vi "Строка параметров в I8 (SubVI).vi"(8 "Строка чисел параметров мишеней":string) -> (9 "Остаток строки":string, 16 "Кластер чисел типа I8":T1)   [LabVIEW 2013]
doc: "Преобразование строки с числами в знаковые байты"
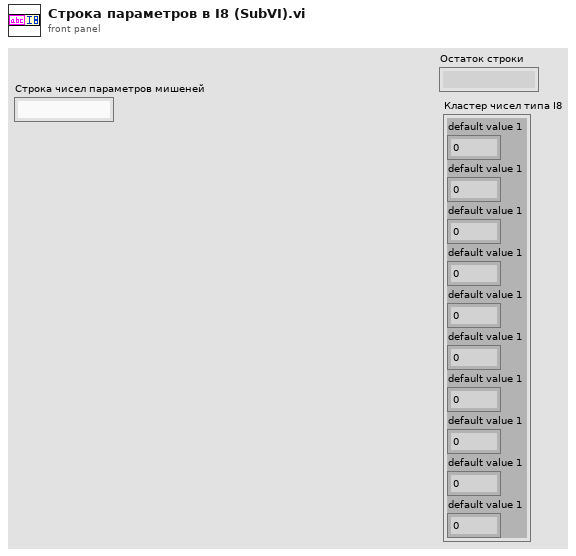
[diagram p1: front panel]
types:
  T1 = cluster{"default value 1":i8, "default value 1":i8, "default value 1":i8, "default value 1":i8, "default value 1":i8, "default value 1":i8, "default value 1":i8, "default value 1":i8, "default value 1":i8, "default value 1":i8}
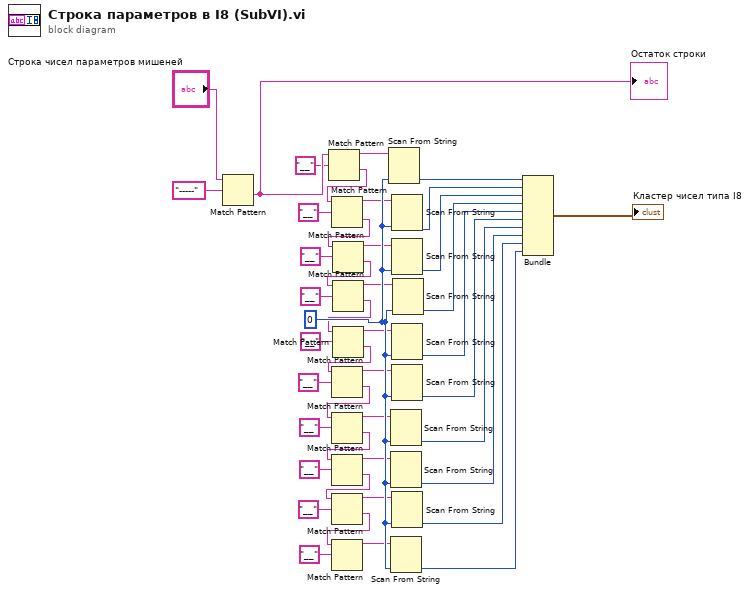
[diagram p0: block diagram]
diagram:
  w44 = i8 0 ("default value 1")
  n1 = Match Pattern(string="Строка чисел параметров мишеней", regular expression="-----") -> (after substring=w40:string)  [unwired: 1 in, 3 out]
  "Остаток строки" <- w40
  n2 = Match Pattern(string=w40, regular expression="__" ("delimiter (Tab)")) -> (before substring=w4:string, after substring=w3:string)  [unwired: 1 in, 2 out]
  n3 = Match Pattern(string=w3, regular expression="__" ("delimiter (Tab)")) -> (before substring=w10:string, after substring=w8:string)  [unwired: 1 in, 2 out]
  n4 = Match Pattern(string=w8, regular expression="__" ("delimiter (Tab)")) -> (before substring=w36:string, after substring=w12:string)  [unwired: 1 in, 2 out]
  n5 = Match Pattern(string=w12, regular expression="__" ("delimiter (Tab)")) -> (before substring=w37:string, after substring=w34:string)  [unwired: 1 in, 2 out]
  n6 = Match Pattern(string=w34, regular expression="__" ("delimiter (Tab)")) -> (before substring=w17:string, after substring=w18:string)  [unwired: 1 in, 2 out]
  n7 = Match Pattern(string=w18, regular expression="__" ("delimiter (Tab)")) -> (before substring=w19:string, after substring=w15:string)  [unwired: 1 in, 2 out]
  n8 = Match Pattern(string=w15, regular expression="__" ("delimiter (Tab)")) -> (before substring=w20:string, after substring=w29:string)  [unwired: 1 in, 2 out]
  n9 = Match Pattern(string=w29, regular expression="__" ("delimiter (Tab)")) -> (before substring=w28:string, after substring=w23:string)  [unwired: 1 in, 2 out]
  n10 = Match Pattern(string=w23, regular expression="__" ("delimiter (Tab)")) -> (before substring=w1:string, after substring=w25:string)  [unwired: 1 in, 2 out]
  n11 = Match Pattern(string=w25, regular expression="__" ("delimiter (Tab)")) -> (before substring=w30:string)  [unwired: 1 in, 3 out]
  n12 = Scan From String(input string=w4, default 1=w44) -> (output 1=w2:i8)  [unwired: 3 in, 3 out]
  n13 = Scan From String(input string=w20, default 1=w44) -> (output 1=w22:i8)  [unwired: 3 in, 3 out]
  n14 = Scan From String(input string=w28, default 1=w44) -> (output 1=w31:i8)  [unwired: 3 in, 3 out]
  n15 = Scan From String(input string=w30, default 1=w44) -> (output 1=w33:i8)  [unwired: 3 in, 3 out]
  n16 = Scan From String(input string=w10, default 1=w44) -> (output 1=w7:i8)  [unwired: 3 in, 3 out]
  n17 = Scan From String(input string=w36, default 1=w44) -> (output 1=w38:i8)  [unwired: 3 in, 3 out]
  n18 = Scan From String(input string=w17, default 1=w44) -> (output 1=w13:i8)  [unwired: 3 in, 3 out]
  n19 = Scan From String(input string=w19, default 1=w44) -> (output 1=w21:i8)  [unwired: 3 in, 3 out]
  n20 = Scan From String(input string=w1, default 1=w44) -> (output 1=w32:i8)  [unwired: 3 in, 3 out]
  n21 = Scan From String(input string=w37, default 1=w44) -> (output 1=w39:i8)  [unwired: 3 in, 3 out]
  n22 = Bundle("default value 1"=w2, "default value 1"=w7, "default value 1"=w38, "default value 1"=w39, "default value 1"=w13, "default value 1"=w21, "default value 1"=w22, "default value 1"=w31, "default value 1"=w32, "default value 1"=w33) -> (→"Кластер чисел типа I8":T1)  [unwired: 1 in]
